vi "update.vi"(8 "error in (no error)":errorcluster, 11 "TrajectoryRK110916Throughput in":refnum<class "TrajectoryRK110916Throughput.lvclass">) -> (0 "error out":errorcluster, 3 "TrajectoryRK110916Throughput out":refnum<class "TrajectoryRK110916Throughput.lvclass">)   [LabVIEW 2010, in "TrajectoryRK110916Throughput.lvclass"]
uses:
  TrajectoryRK110916Throughput.lvclass
  FPGAWrapper/GenericFPGAWrapper/GenericFPGAWrapper/GenericFPGAWrapper.lvclass
  FPGAWrapper/FPGAWrapperRK110909Throughput/FPGAWrapperRK110909Throughput/FPGAWrapperRK110909Throughput.lvclass
  TrajectoryRK110916Throughput.lvclass/TrajectoryRK110916Throughput.ctl
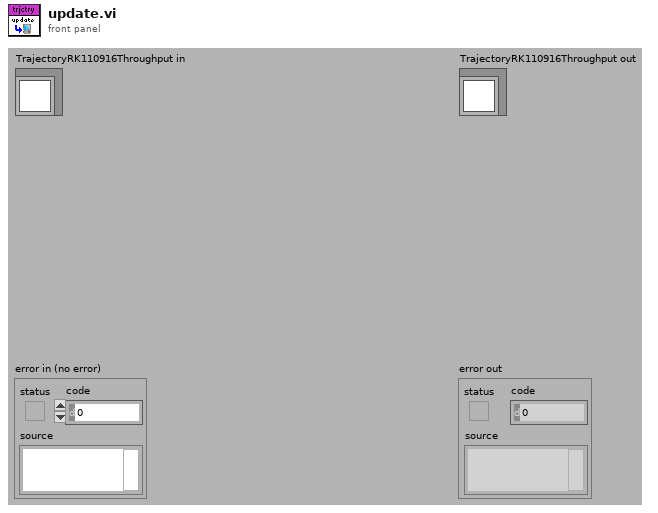
[diagram p1: front panel]
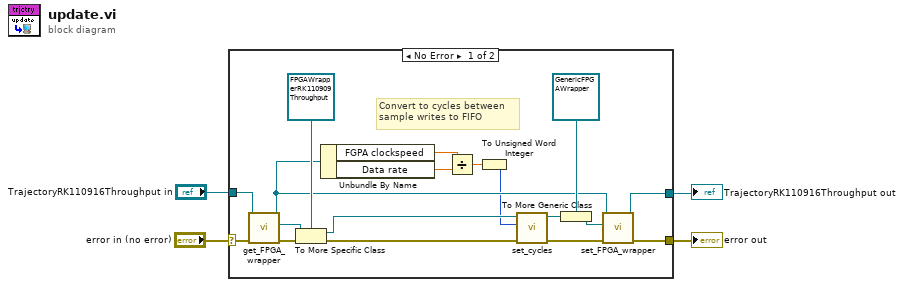
[diagram p0: block diagram]
diagram:
  n1 = case shown="No Error" "error in (no error)" {
    selector: "error in (no error)" -> [w22 w23]
    tunnel: [w12 w23] -> w3
    tunnel: [w9 w24] -> w1
    tunnel: "TrajectoryRK110916Throughput in" -> [w21 w24]
    frame No Error {
      # "Convert to cycles between\nsample writes to FIFO"
      n2 = call-dynamic "get_FPGA_wrapper.vi"("error in (no error)"=w22, "TrajectoryMG100122GenericFPGA in"=w21) -> ("error out"=w20:errorcluster, "GenericFPGAWrapper.lvclass"=w18:refnum<class "GenericFPGAWrapper.lvclass">, "TrajectoryMG100122GenericFPGA out"=w10:refnum<class "TrajectoryRK110916Throughput.lvclass">)  [unwired: 7 in]
      n3 = To More Specific Class(target class=refnum<class "FPGAWrapperRK110909Throughput.lvclass"> refnum ("FPGAWrapperRK110909Throughput.lvclass"), reference=w18, error in=w20) -> (specific class reference=w16:refnum<class "FPGAWrapperRK110909Throughput.lvclass">, error out=w19:errorcluster)
      n4 = Unbundle By Name(w10) -> ("FGPA clockspeed"=w8:dbl, "Data rate"=w7:dbl)
      n5 = Divide(x=w8, y=w7) -> (x/y=w6:dbl)
      n6 = To Unsigned Word Integer(number=w6) -> (unsigned 16bit integer=w5:u16)
      n7 = call "set_cycles.vi"("error in"=w19, "Cycles"=w5, "FPGAWrapperRK110909Throughput in"=w16) -> ("error out"=w13:errorcluster, "FPGAWrapperRK110909Throughput in 2"=w15:refnum<class "FPGAWrapperRK110909Throughput.lvclass">)  [unwired: 7 in]
      n8 = To More Generic Class(target class=refnum<class "GenericFPGAWrapper.lvclass"> refnum ("GenericFPGAWrapper.lvclass"), reference=w15) -> (generic class reference=w11:refnum<class "GenericFPGAWrapper.lvclass">)
      n9 = call-dynamic "set_FPGA_wrapper.vi"("error in (no error)"=w13, "GenericFPGAWrapper.lvclass"=w11, "TrajectoryMG100122GenericFPGA in"=w10) -> ("error out"=w12:errorcluster, "TrajectoryMG100122GenericFPGA out"=w9:refnum<class "TrajectoryRK110916Throughput.lvclass">)  [unwired: 7 in]
    }
    frame Error {
    }
  }
  "error out" <- w3
  "TrajectoryRK110916Throughput out" <- w1
